vi "Pre Launch Init.vi"(11 "Customer in":refnum<class "Customer.lvclass">) -> (0 "error out":errorcluster, 3 "Customer out":refnum<class "Customer.lvclass">)   [LabVIEW 2023, in "Customer.lvlib" / "Customer.lvclass"]
doc: "(<B>Filename</B>: Actor Framework.lvlib:Actor.lvclass:Pre Launch Init.vi)\n\nDefines behavior that occurs after the Launch Nested Actor method is invoked but before the actor's Actor Core method begins running.\n\nBy default, this method does nothing. A descendant class may override it to define behavior."
uses:
  Customer.lvclass
  Customer.lvclass/Customer.ctl
  Person/Person.lvclass
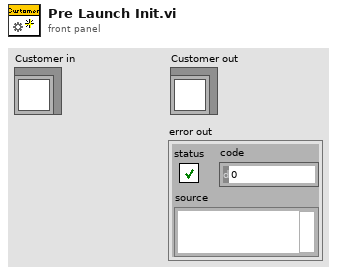
[diagram p1: front panel]
types:
  T1 = cluster{"Item":refnum<user-event>, "Order #":refnum<user-event>, "Stop":refnum<user-event>}
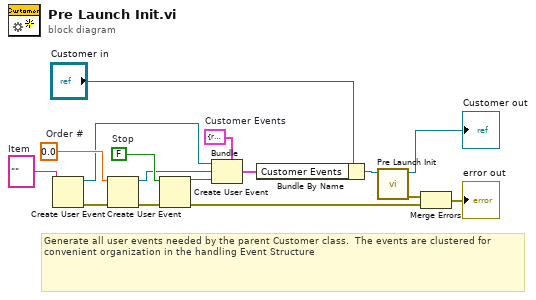
[diagram p0: block diagram]
diagram:
  w4 = T1 {"Item"=refnum, "Order #"=refnum, "Stop"=refnum}  # Customer Events
  w11 = ""  # Item
  w13 = 0.0  # Order #
  w15 = FALSE  # Stop
  # "Generate all user events needed by the parent Customer class.  The events are clustered for convenient organization in the handling Event Structure"
  n1 = Create User Event(user event datatype=w11) -> (user event=w7:refnum<user-event>, error out=w12:errorcluster)  [unwired: 1 in]
  n2 = Create User Event(user event datatype=w13, error in=w12) -> (user event=w6:refnum<user-event>, error out=w14:errorcluster)
  n3 = Create User Event(user event datatype=w15, error in=w14) -> (user event=w5:refnum<user-event>, error out=w9:errorcluster)
  n4 = Bundle(cluster=w4, "Item"=w7, "Order #"=w6, "Stop"=w5) -> (w1:T1)
  n5 = Bundle By Name(cluster="Customer in", "Customer Events"=w1) -> (w2:refnum<class "Customer.lvclass">)
  n6 = call-parent "Pre Launch Init.vi"("Person in"=w2) -> ("error out"=w10:errorcluster, "Person out"=→"Customer out":refnum<class "Customer.lvclass">)  [unwired: 9 in]
  n7 = Merge Errors(w10, w9) -> (→"error out":errorcluster)
